vi "sid_prbs.vi"() -> (0 "Init Data Out":bool[](array[boolean]))   [LabVIEW 2016]
panel:
  # "For Initialization VI requirements and help, please read directions located on Block Diagram."
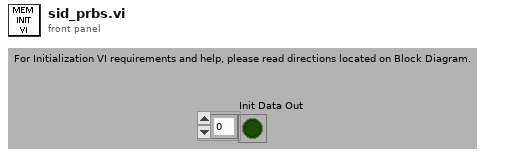
[diagram p1: front panel]
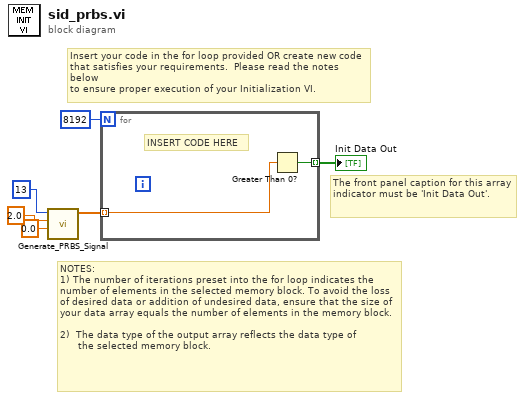
[diagram p0: block diagram]
diagram:
  # "The front panel caption for this array indicator must be 'Init Data Out'."
  # "NOTES:\n1) The number of iterations preset into the for loop indicates the number of elements in the selected memory block. To avoid the loss of desired data or addition of undesired data, ensure that the size of your data array equals the number of elements in the memory block.\n\n2)  The data type of the output array reflects the data type of\n      the selected memory block."
  # "Insert your code in the for loop provided OR create new code\nthat satisfies your requirements.  Please read the notes below\nto ensure proper execution of your Initialization VI."
  n1 = call "Generate_PRBS_Signal.vi"("Min.Value"=0.0, "Max. Value"=2.0, "PRBS Order"=13) -> ("PRBS Signal"=w1:dbl[])  [unwired: 7 in, 1 out]
  n2 = for {
    N: 8192 ("Number of Elements") -> [_]
    tunnel: [w8] -> w5 mode=indexing
    tunnel: w1 -> [w7] mode=indexing
    # "INSERT CODE HERE"
    n3 = Greater Than 0?(x=w7) -> (x > 0?=w8:bool)
  }
  "Init Data Out" <- w5
